vi "Page_Source_Settings_Update_Display.vi"(6 "AB_Build in":refnum<class "AB_Build.lvclass">, 8 "error in (no error)":errorcluster, 9 "ctlReferences":T3, 10 "supportedFunctions":T2, 11 "AB_Source_Container in":refnum<class "AB_Source_Container.lvclass">) -> (0 "error out":errorcluster, 2 "parentApplies":T1, 3 "AB_Source_Container out":refnum<class "AB_Source_Container.lvclass">)   [LabVIEW 2020, in "AB_Source_Container.lvclass"]
uses:
  <vilib>/AppBuilder/AB_Classes/Source/Container/AB_Source_Container.lvclass
  e:/builds/penguin/labview/branches/2020/dev/dist/vi.lib/AppBuilder/AB_Classes/Source/AB_Source.lvclass
  <resource>/Framework/Providers/Builds/AppBuilder/AB_UI_Page_Source_Settings_References.ctl
  <resource>/Framework/Providers/Builds/AppBuilder/AB_UI_Page_Source_Settings_supportedFunctions.ctl
  <vilib>/AppBuilder/AB_Parent_Applies.ctl
  <vilib>/AppBuilder/AB_Classes/Build/AB_Build.lvclass
  <vilib>/AppBuilder/AB_Source_Inclusion.ctl
  <resource>/Framework/Providers/Common/provcom_StringGlobals.vi
  <vilib>/AppBuilder/AB_Classes/Source/AB_Source.lvclass
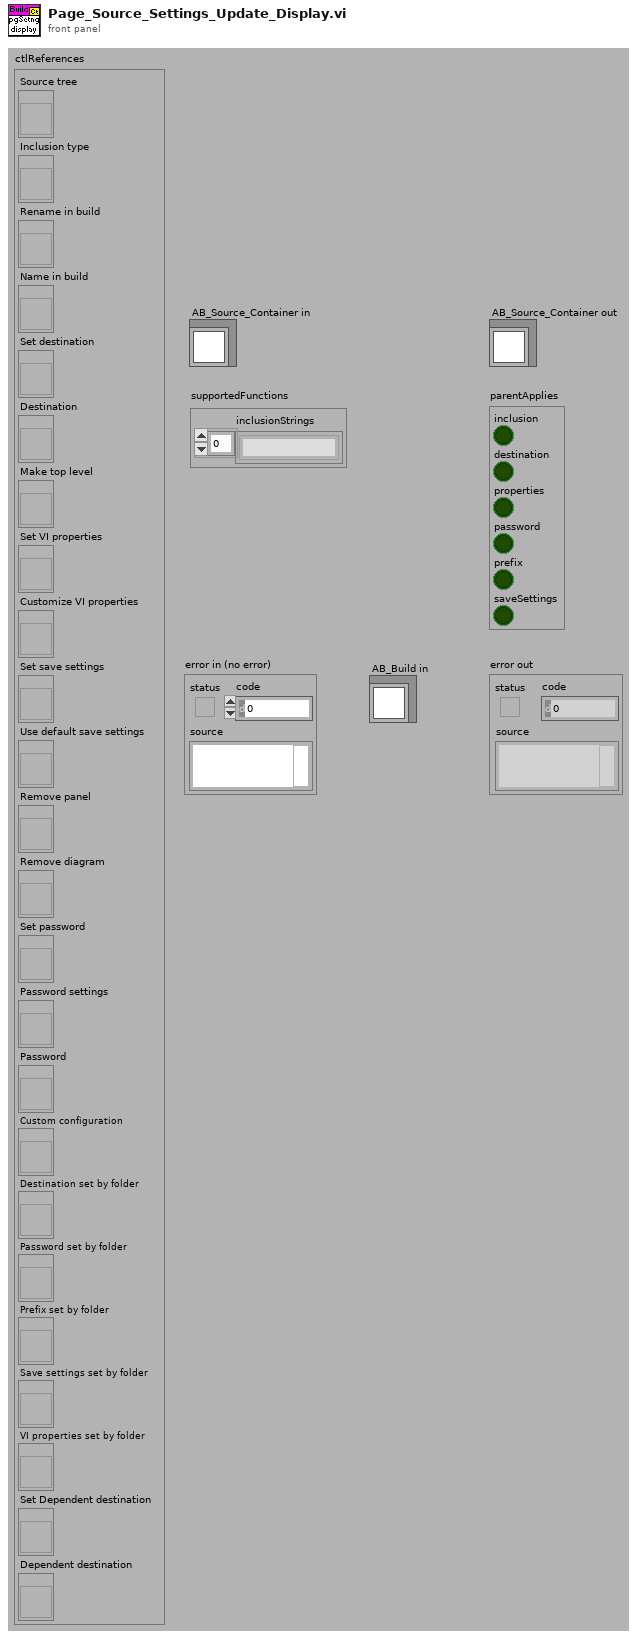
[diagram p1: front panel]
types:
  T1 = typedef "AB_Parent_Applies.ctl" = cluster{"inclusion":bool, "destination":bool, "properties":bool, "password":bool, "prefix":bool, "saveSettings":bool}
  T2 = typedef "AB_UI_Page_Source_Settings_supportedFunctions.ctl" = cluster{"inclusionStrings":string[]}
  T3 = typedef "AB_UI_Page_Source_Settings_References.ctl" = cluster{"Source tree":refnum<vi>, "Inclusion type":refnum<vi>, "Rename in build":refnum<vi>, "Name in build":refnum<vi>, "Set destination":refnum<vi>, "Destination":refnum<vi>, "Make top level":refnum<vi>, "Set VI properties":refnum<vi>, "Customize VI properties":refnum<vi>, "Set save settings":refnum<vi>, "Use default save settings":refnum<vi>, "Remove panel":refnum<vi>, "Remove diagram":refnum<vi>, "Set password":refnum<vi>, "Password settings":refnum<vi>, "Password":refnum<vi>, "Custom configuration":refnum<vi>, "Destination set by folder":refnum<vi>, "Password set by folder":refnum<vi>, "Prefix set by folder":refnum<vi>, "Save settings set by folder":refnum<vi>, "VI properties set by folder":refnum<vi>, "Set Dependent destination":refnum<vi>, "Dependent destination":refnum<vi>}
  T4 = typedef "AB_Build.ctl" = cluster{"buildSpecName":string, "buildSpecDescription":string, "destinations":refnum<class "AB_Destination.lvclass">[], "exclusionOption":T5, "defaultLanguage":string, "supportedLanguages":string[], "excludedDirectories":path[], "buildContext":refnum<vi>, "buildObject":T6, "preview":bool, "programatic":bool, "progressBarEvents":T7, "userLog_Path":path, "preActionID":string, "preAction_Path":path, "postActionID":string, "postAction_Path":path, "eng_checkForBrokenVIs?":bool, "eng_verboseLinkerErrors?":bool, "localDest_Path":path, "targetDest_Path":path, "removeVIObject":u16, "cache":refnum<class "PreviewCache.lvclass">, "use cache":bool, "previewCache_ID":string, "buildCache_ID":string, "eng_TempLocalDest_Path":path, "eng_collectDependencies?":bool, "versionInfo":cluster{"buildVersion":cluster{"major":u16, "minor":u16, "patch":u16, "build":u16}, "autoIncrement":bool}, "eng_enableVIChecksums":bool}
  T5 = typedef "AB_Exclusion_Option.ctl" = cluster{"typedefs":bool, "polymorphicVIs":bool, "unusedLibraryItems":bool, "modifyLibraryFile":bool, "edit-timeDependencies":bool, "inlineVIs":bool, "dependent PPLs":bool, "dependent DLLs":bool}
  T6 = typedef "ItemRef.ctl" = u64
  T7 = typedef "provcom_ProgressBar_Events.ctl" = cluster{"newJob":refnum<user-event>, "newItem":refnum<user-event>, "errorMsg":T8, "cancel":refnum<user-event>}
  T8 = typedef "mxLvBuildError.ctl" = refnum<user-event>
  T9 = typedef "AB_Source.ctl" = cluster{"path":path, "itemID":string, "parentIndex":i32, "sourceInclusion":T10, "destinationIndex":i32, "properties":T11[], "newName":string, "lvfile":bool, "valid":bool, "eng_inBuild":bool, "eng_isNonVILink":bool, "Amalgamation":bool, "Amalgamation Piece":bool, "eng_delimitedName":string, "preventRename":bool}
  T10 = typedef "AB_Source_Inclusion.ctl" = enum16{"IncludeIfReferenced", "Include", "Exclude", "TopLevel"}
  T11 = typedef "AB_Source_Properties.ctl" = cluster{"sourcePropertyType":T12, "value":variant}
  T12 = typedef "AB_Source_Property_Type.ctl" = enum16{"Remove block diagram", "Remove front panel", "Password", "Window has title bar", "Show menu bar", "Show vertical scroll bar", "Show horizontal scroll bar", "Show toolbar", "Show Abort button", "Show fp when called", "Window behavior", "Allow user to close window", "Window run-time position", "Run when opened", "Allow debugging", "Auto error handling", "Generate guard code", "Use stack variables", "Expression folding", "Integer only", "Inline subVI"}
  T13 = typedef "AB_Source_Container.ctl" = cluster{"applyInclusion":bool, "applyDestination":bool, "applyProperties":bool, "applyPassword":bool, "applyPrefix":bool, "applySaveSetttings":bool, "dependentDestinationIndex":i32}
  T14 = enum32{"No password change", "Remove password", "Apply new password"}
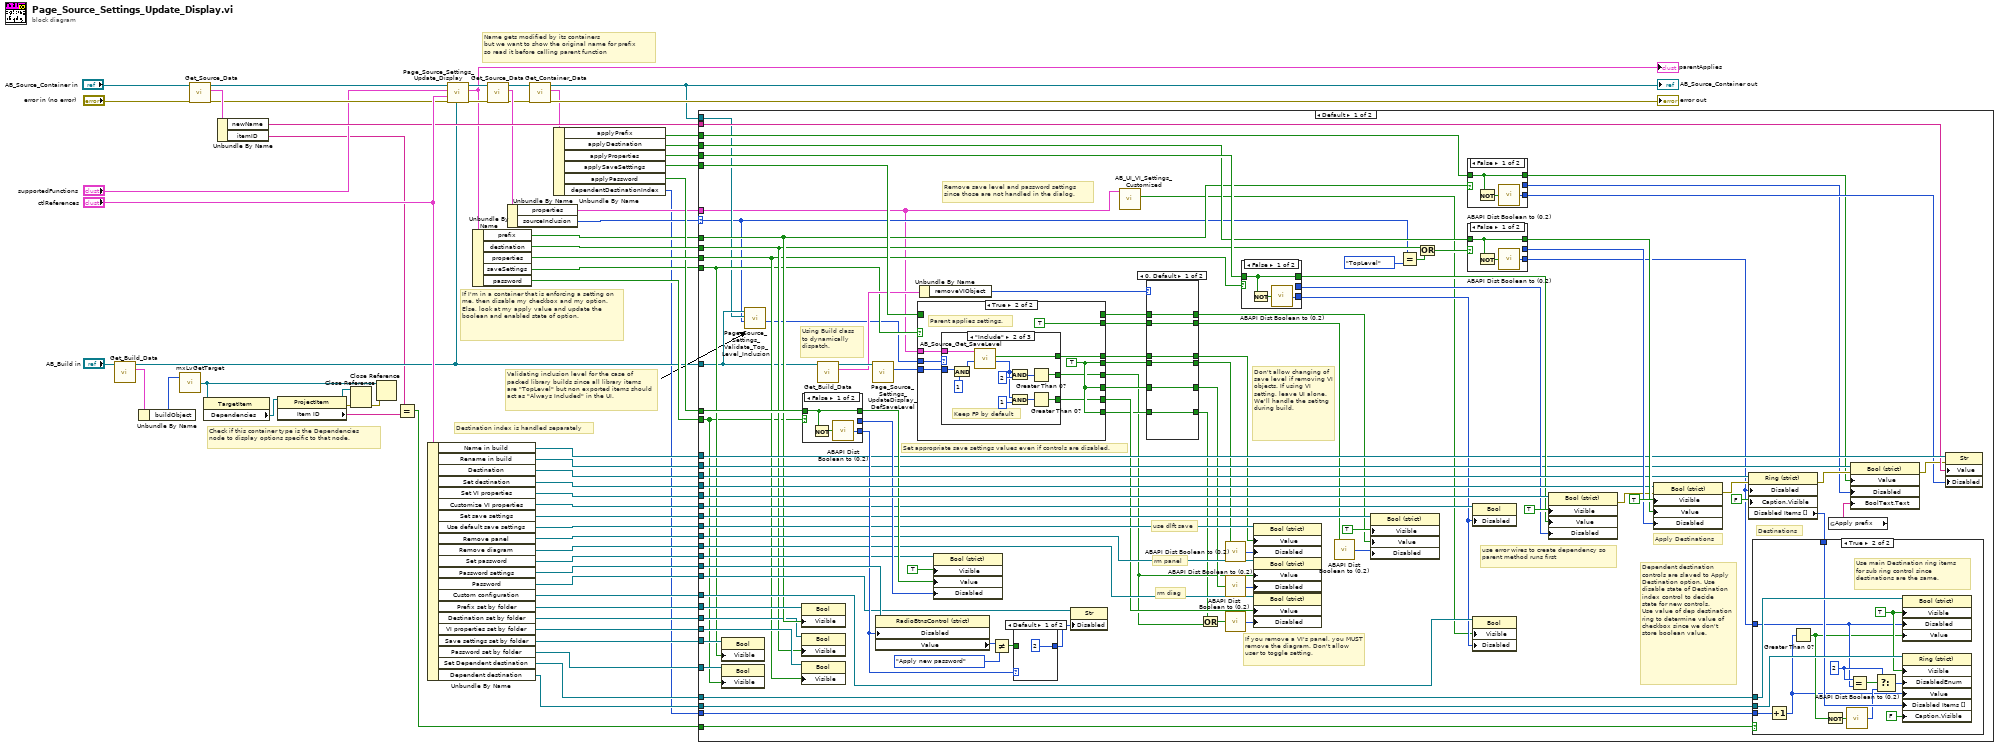
[diagram p0: block diagram]
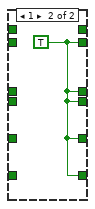
[diagram p3: hidden frame]
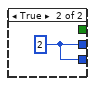
[diagram p4: hidden frame]
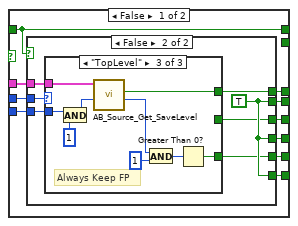
[diagram p5: hidden frame]
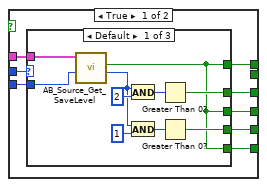
[diagram p6: hidden frame]
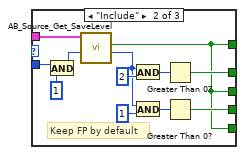
[diagram p7: hidden frame]
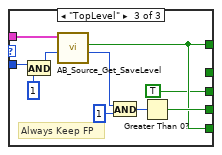
[diagram p8: hidden frame]
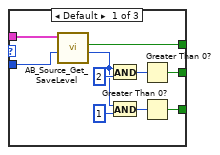
[diagram p9: hidden frame]
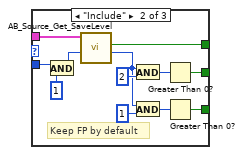
[diagram p10: hidden frame]
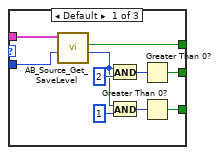
[diagram p11: hidden frame]
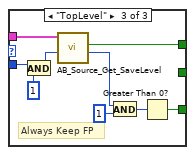
[diagram p12: hidden frame]
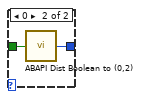
[diagram p13: hidden frame]
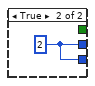
[diagram p14: hidden frame]
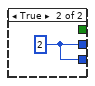
[diagram p15: hidden frame]
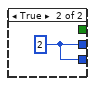
[diagram p16: hidden frame]
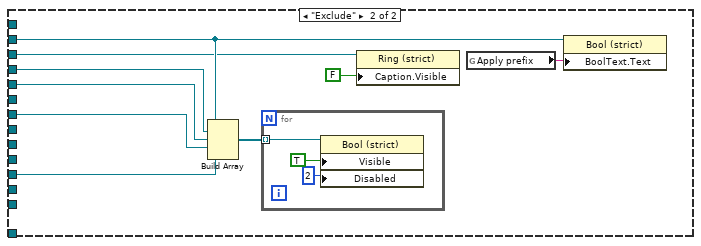
[diagram p17: hidden frame]
diagram:
  # "Check if this container type is the Dependencies node to display options specific to that node."
  # "Validating inclusion level for the case of packed library builds since all library items are \"TopLevel\" but non exported items should act as \"Always Included\" in the UI."
  # "If I'm in a container that is enforcing a setting on me, then disable my checkbox and my option.\nElse, look at my apply value and update the boolean and enabled state of option."
  # "Name gets modified by its containers\nbut we want to show the original name for prefix\nso read it before calling parent function"
  # "Destination index is handled separately"
  n1 = call <vilib>:"Get_Build_Data.vi"("Class in"="AB_Build in") -> ("data"=w12:T4, "Class out"=w13:refnum<class "AB_Build.lvclass">)  [unwired: 8 in, 1 out]
  n2 = Unbundle By Name(w12) -> ("buildObject"=w6:T6)
  n3 = call <resource>:"mxLvGetTarget.vi"("Item"=w6) -> ("Target"=w7:refnum<vi>)  [unwired: 1 in, 2 out]
  n4 = call <vilib>:"Get_Source_Data.vi"("error in (no error)"="error in (no error)", "Class in"="AB_Source_Container in") -> ("error out"=w47:errorcluster, "data"=w51:T9, "Class out"=w49:refnum<class "AB_Source_Container.lvclass">)  [unwired: 7 in]
  n5 = property class="TargetItem"(reference=w7) -> ("Dependencies"=w11:refnum<vi>)  [unwired: 1 in, 2 out]
  n6 = Unbundle By Name(w51) -> ("newName"=w50:string, "itemID"=w4:string)
  n7 = property class="ProjectItem"(reference=w11) -> (reference out=w9:refnum<vi>, error out=w10:errorcluster, "Item ID"=w5:string)  [unwired: 1 in]
  n8 = Close Reference(reference=w9, error in (no error)=w10) -> (error out=w8:errorcluster)
  n9 = Close Reference(reference=w7, error in (no error)=w8) -> ()  [unwired: 1 out]
  n10 = Equal?(x=w4, y=w5) -> (x = y?=w3:bool)
  n11 = Unbundle By Name("ctlReferences") -> ("Name in build"=w53:refnum<vi>, "Rename in build"=w54:refnum<vi>, "Destination"=w59:refnum<vi>, "Set destination"=w61:refnum<vi>, "Set VI properties"=w60:refnum<vi>, "Customize VI properties"=w34:refnum<vi>, "Set save settings"=w33:refnum<vi>, "Use default save settings"=w32:refnum<vi>, "Remove panel"=w28:refnum<vi>, "Remove diagram"=w27:refnum<vi>, "Set password"=w35:refnum<vi>, "Password settings"=w62:refnum<vi>, "Password"=w58:refnum<vi>, "Custom configuration"=w23:refnum<vi>, "Prefix set by folder"=w22:refnum<vi>, "Destination set by folder"=w21:refnum<vi>, "VI properties set by folder"=w20:refnum<vi>, "Save settings set by folder"=w19:refnum<vi>, "Password set by folder"=w18:refnum<vi>, "Set Dependent destination"=w16:refnum<vi>, "Dependent destination"=w15:refnum<vi>)
  n12 = call-parent "Page_Source_Settings_Update_Display.vi"("AB_Build in"=w13, "error in (no error)"=w47, "ctlReferences"="ctlReferences", "supportedFunctions"="supportedFunctions", "AB_Source in"=w49) -> ("error out"=w43:errorcluster, "parentApplies"=w1:T1, "AB_Source out"=w45:refnum<class "AB_Source_Container.lvclass">)  [unwired: 4 in]
  "parentApplies" <- w1
  n13 = Unbundle By Name(w1) -> ("prefix"=w24:bool, "destination"=w57:bool, "properties"=w56:bool, "saveSettings"=w30:bool, "password"=w55:bool)
  n14 = call <vilib>:"Get_Source_Data.vi"("error in (no error)"=w43, "Class in"=w45) -> ("error out"=w42:errorcluster, "data"=w46:T9, "Class out"=w44:refnum<class "AB_Source_Container.lvclass">)  [unwired: 7 in]
  n15 = Unbundle By Name(w46) -> ("properties"=w29:T11[], "sourceInclusion"=w25:T10)
  n16 = call <vilib>:"Get_Container_Data.vi"("error in (no error)"=w42, "Class in"=w44) -> ("error out"=→"error out":errorcluster, "data"=w40:T13, "Class out"=w17:refnum<class "AB_Source_Container.lvclass">)  [unwired: 7 in]
  "AB_Source_Container out" <- w17
  n17 = Unbundle By Name(w40) -> ("applyPrefix"=w36:bool, "applyDestination"=w37:bool, "applyProperties"=w38:bool, "applySaveSetttings"=w26:bool, "applyPassword"=w39:bool, "dependentDestinationIndex"=w2:i32)
  n18 = case shown="Default" w25 {
    selector: w25 -> [w73 _]
    tunnel: w62 -> [w156 _]
    tunnel: w61 -> [w152 w329]
    tunnel: w60 -> [w149 w330]
    tunnel: w59 -> [w148 w324]
    tunnel: w58 -> [w141 _]
    tunnel: w57 -> [w85 _]
    tunnel: w56 -> [w84 _]
    tunnel: w55 -> [w80 _]
    tunnel: w54 -> [w133 w328]
    tunnel: w53 -> [w132 _]
    tunnel: w50 -> [w131 _]
    tunnel: w39 -> [w130 _]
    tunnel: w38 -> [w129 _]
    tunnel: w37 -> [w128 _]
    tunnel: w36 -> [w108 _]
    tunnel: w35 -> [w123 w327]
    tunnel: w34 -> [w122 _]
    tunnel: w33 -> [w120 w331]
    tunnel: w32 -> [w119 _]
    tunnel: w30 -> [w81 _]
    tunnel: w29 -> [w71 _]
    tunnel: w28 -> [w118 _]
    tunnel: w27 -> [w117 _]
    tunnel: w26 -> [w113 _]
    tunnel: w24 -> [w88 _]
    tunnel: w13 -> [w75 _]
    tunnel: w23 -> [w91 _]
    tunnel: w22 -> [w89 _]
    tunnel: w21 -> [w87 _]
    tunnel: w20 -> [w86 _]
    tunnel: w19 -> [w83 _]
    tunnel: w18 -> [w82 _]
    tunnel: w17 -> [w74 _]
    tunnel: w16 -> [w68 _]
    tunnel: w15 -> [w67 _]
    tunnel: w3 -> [w69 _]
    tunnel: w2 -> [w65 _]
    frame Default {
      # "Dependent destination controls are slaved to Apply Destination option. Use disable state of Destination index control to decide state for new controls. \nUse value of dep destination ring to determine value of checkbox since we don't store boolean value."
      # "Apply Destinations"
      # "Destinations"
      # "Remove save level and password settings since those are not handled in the dialog."
      # "Set appropriate save settings values even if controls are disabled."
      # "use dlft save"
      # "rm diag"
      # "rm panel"
      # "If you remove a VI's panel, you MUST remove the diagram. Don't allow user to toggle setting."
      # "Don't allow changing of save level if removing VI objects. If using VI setting, leave UI alone. We'll handle the setitng during build."
      # "Using Build class to dynamically dispatch."
      # "use error wires to create dependency so parent method runs first"
      n19 = property class="Bool"(reference=w83, "Visible"=w81) -> ()  [unwired: 1 in, 2 out]
      n20 = property class="Bool"(reference=w82, "Visible"=w80) -> ()  [unwired: 1 in, 2 out]
      n21 = call-dynamic "Page_Source_Settings_Validate_Top_Level_Inclusion.vi"("sourceInclusion in"=w73, "AB_Source in"=w74, "AB_Build in"=w75) -> ("sourceInclusion out"=w72:T10)  [unwired: 6 in, 2 out]
      n22 = property class="Bool"(reference=w89, "Visible"=w88) -> ()  [unwired: 1 in, 2 out]
      n23 = property class="Bool"(reference=w87, "Visible"=w85) -> ()  [unwired: 1 in, 2 out]
      n24 = property class="Bool"(reference=w86, "Visible"=w84) -> ()  [unwired: 1 in, 2 out]
      n25 = case shown="False" w80 {
        tunnel: [_ w315] -> w144
        tunnel: [w314 _] -> w145
        tunnel: w130 -> [w314 _]
        tunnel: [w312 w315] -> w142
        frame False {
          n26 = Not(x=w314) -> (.not. x?=w313:bool)
          n27 = call <vilib>:"ABAPI Dist Boolean to (0,2).vi"("Boolean"=w313) -> ("0, 2"=w312:u8)  [unwired: 4 in]
        }
        frame True {
          w315 = u8 2 ("Disabled")
        }
      }
      n28 = call <vilib>:"Get_Build_Data.vi"("Class in"=w75) -> ("data"=w104:T4, "Class out"=w105:refnum<class "AB_Build.lvclass">)  [unwired: 8 in, 1 out]
      n29 = call-dynamic "Page_Source_Settings_UpdateDisplay_DefSaveLevel.vi"("AB_Build in"=w105) -> ("defaultSaveLevel"=w106:u32)  [unwired: 8 in, 2 out]
      n30 = property class="RadioBtnsControl (strict)"(reference=w156, "Disabled"=w142) -> ("Value"=w140:T14)  [unwired: 1 in, 2 out]
      n31 = case shown="True" w81 {
        tunnel: w106 -> [w191 w271]
        tunnel: w71 -> [w190 w270]
        tunnel: [w188 w273] -> w102
        tunnel: [w187 w277] -> w101
        tunnel: [w186 w275] -> w79
        tunnel: [w185 w277] -> w100
        tunnel: [w184 w274] -> w114
        tunnel: [w183 w277] -> w99
        tunnel: w113 -> [w182 _]
        tunnel: w72 -> [w189 w272]
        tunnel: [w182 _] -> w95
        tunnel: [_ TRUE] -> w94
        frame False {
          n32 = case shown="False" w182 {
            tunnel: w189 -> [w192 w234]
            tunnel: w190 -> [w199 w233]
            tunnel: [w198 w235] -> w188
            tunnel: [_ w238] -> w187
            tunnel: [w197 w238] -> w185
            tunnel: [w196 w238] -> w183
            tunnel: w191 -> [w195 w232]
            tunnel: [w194 w237] -> w186
            tunnel: [w193 w236] -> w184
            frame True {
              n33 = case shown="Default" w192 {
                tunnel: w199 -> [w209 w221 w231]
                tunnel: [w200 w210 w227] -> w198
                tunnel: [w200 w210 TRUE] -> w197
                tunnel: [w200 w210 w227] -> w196
                tunnel: w195 -> [w208 w216 w225]
                tunnel: [w205 w212 _] -> w194
                tunnel: [w201 w218 w228] -> w193
                frame Default {
                  n34 = call <vilib>:"AB_Source_Get_SaveLevel.vi"("defaultSaveLevel"=w208, "sourceProperties in"=w209) -> ("saveLevel out"=w202:u32, "useDefault"=w200:bool)  [unwired: 6 in, 2 out]
                  n35 = And(x=w202, y=u32 2) -> (x .and. y?=w206:u32)
                  n36 = And(x=w202, y=u32 1) -> (x .and. y?=w204:u32)
                  n37 = Greater Than 0?(x=w206) -> (x > 0?=w205:bool)
                  n38 = Greater Than 0?(x=w204) -> (x > 0?=w201:bool)
                }
                frame "Include" {
                  # "Keep FP by default"
                  n39 = And(x=w216, y=u32 1 ("defaultSaveLevel")) -> (x .and. y?=w215:u32)
                  n40 = call <vilib>:"AB_Source_Get_SaveLevel.vi"("defaultSaveLevel"=w215, "sourceProperties in"=w221) -> ("saveLevel out"=w211:u32, "useDefault"=w210:bool)  [unwired: 6 in, 2 out]
                  n41 = And(x=w211, y=u32 2) -> (x .and. y?=w213:u32)
                  n42 = And(x=w211, y=u32 1) -> (x .and. y?=w220:u32)
                  n43 = Greater Than 0?(x=w213) -> (x > 0?=w212:bool)
                  n44 = Greater Than 0?(x=w220) -> (x > 0?=w218:bool)
                }
                frame "TopLevel" {
                  # "Always Keep FP"
                  n45 = And(x=w225, y=u32 1 ("defaultSaveLevel")) -> (x .and. y?=w224:u32)
                  n46 = call <vilib>:"AB_Source_Get_SaveLevel.vi"("defaultSaveLevel"=w224, "sourceProperties in"=w231) -> ("saveLevel out"=w223:u32, "useDefault"=w227:bool)  [unwired: 6 in, 2 out]
                  n47 = And(x=w223, y=u32 1) -> (x .and. y?=w230:u32)
                  n48 = Greater Than 0?(x=w230) -> (x > 0?=w228:bool)
                }
              }
            }
            frame False {
              w238 = TRUE
              n49 = case shown="\"TopLevel\"" w234 {
                tunnel: w233 -> [w248 w260 w269]
                tunnel: [w239 w249 w261] -> w235
                tunnel: w232 -> [w247 w255 w264]
                tunnel: [w244 w251 _] -> w237
                tunnel: [w240 w257 w266] -> w236
                frame Default {
                  n50 = call <vilib>:"AB_Source_Get_SaveLevel.vi"("defaultSaveLevel"=w247, "sourceProperties in"=w248) -> ("saveLevel out"=w241:u32, "useDefault"=w239:bool)  [unwired: 6 in, 2 out]
                  n51 = And(x=w241, y=u32 2) -> (x .and. y?=w245:u32)
                  n52 = And(x=w241, y=u32 1) -> (x .and. y?=w243:u32)
                  n53 = Greater Than 0?(x=w245) -> (x > 0?=w244:bool)
                  n54 = Greater Than 0?(x=w243) -> (x > 0?=w240:bool)
                }
                frame "Include" {
                  # "Keep FP by default"
                  n55 = And(x=w255, y=u32 1 ("defaultSaveLevel")) -> (x .and. y?=w254:u32)
                  n56 = call <vilib>:"AB_Source_Get_SaveLevel.vi"("defaultSaveLevel"=w254, "sourceProperties in"=w260) -> ("saveLevel out"=w250:u32, "useDefault"=w249:bool)  [unwired: 6 in, 2 out]
                  n57 = And(x=w250, y=u32 2) -> (x .and. y?=w252:u32)
                  n58 = And(x=w250, y=u32 1) -> (x .and. y?=w259:u32)
                  n59 = Greater Than 0?(x=w252) -> (x > 0?=w251:bool)
                  n60 = Greater Than 0?(x=w259) -> (x > 0?=w257:bool)
                }
                frame "TopLevel" {
                  # "Always Keep FP"
                  n61 = And(x=w264, y=u32 1 ("defaultSaveLevel")) -> (x .and. y?=w263:u32)
                  n62 = call <vilib>:"AB_Source_Get_SaveLevel.vi"("defaultSaveLevel"=w263, "sourceProperties in"=w269) -> ("saveLevel out"=w262:u32, "useDefault"=w261:bool)  [unwired: 6 in, 2 out]
                  n63 = And(x=w262, y=u32 1) -> (x .and. y?=w268:u32)
                  n64 = Greater Than 0?(x=w268) -> (x > 0?=w266:bool)
                }
              }
            }
          }
        }
        frame True {
          w277 = TRUE
          # "Parent applies settings."
          n65 = case shown="\"Include\"" w272 {
            tunnel: w270 -> [w287 w299 w308]
            tunnel: [w278 w288 w300] -> w273
            tunnel: w271 -> [w286 w294 w303]
            tunnel: [w283 w290 _] -> w275
            tunnel: [w279 w296 w305] -> w274
            frame Default {
              n66 = call <vilib>:"AB_Source_Get_SaveLevel.vi"("defaultSaveLevel"=w286, "sourceProperties in"=w287) -> ("saveLevel out"=w280:u32, "useDefault"=w278:bool)  [unwired: 6 in, 2 out]
              n67 = And(x=w280, y=u32 2) -> (x .and. y?=w284:u32)
              n68 = And(x=w280, y=u32 1) -> (x .and. y?=w282:u32)
              n69 = Greater Than 0?(x=w284) -> (x > 0?=w283:bool)
              n70 = Greater Than 0?(x=w282) -> (x > 0?=w279:bool)
            }
            frame "Include" {
              # "Keep FP by default"
              n71 = And(x=w294, y=u32 1 ("defaultSaveLevel")) -> (x .and. y?=w293:u32)
              n72 = call <vilib>:"AB_Source_Get_SaveLevel.vi"("defaultSaveLevel"=w293, "sourceProperties in"=w299) -> ("saveLevel out"=w289:u32, "useDefault"=w288:bool)  [unwired: 6 in, 2 out]
              n73 = And(x=w289, y=u32 2) -> (x .and. y?=w291:u32)
              n74 = And(x=w289, y=u32 1) -> (x .and. y?=w298:u32)
              n75 = Greater Than 0?(x=w291) -> (x > 0?=w290:bool)
              n76 = Greater Than 0?(x=w298) -> (x > 0?=w296:bool)
            }
            frame "TopLevel" {
              # "Always Keep FP"
              n77 = And(x=w303, y=u32 1 ("defaultSaveLevel")) -> (x .and. y?=w302:u32)
              n78 = call <vilib>:"AB_Source_Get_SaveLevel.vi"("defaultSaveLevel"=w302, "sourceProperties in"=w308) -> ("saveLevel out"=w301:u32, "useDefault"=w300:bool)  [unwired: 6 in, 2 out]
              n79 = And(x=w301, y=u32 1) -> (x .and. y?=w307:u32)
              n80 = Greater Than 0?(x=w307) -> (x > 0?=w305:bool)
            }
          }
        }
      }
      n81 = Unbundle By Name(w104) -> ("removeVIObject"=w103:u16)
      n82 = property class="Bool (strict)"(reference=w123, "Visible"=TRUE, "Value"=w145, "Disabled"=w144) -> ()  [unwired: 1 in, 2 out]
      n83 = Not Equal?(x=w140, y=T14."Apply new password") -> (x != y?=w138:bool)
      n84 = case shown="Default" w142 {
        tunnel: w138 -> [_ w311]
        tunnel: [u8 2 ("0, 2") w310] -> w137
        frame Default {
        }
        frame 0 {
          n85 = call <vilib>:"ABAPI Dist Boolean to (0,2).vi"("Boolean"=w311) -> ("0, 2"=w310:u8)  [unwired: 4 in]
        }
      }
      n86 = property class="Str"(reference=w141, "Disabled"=w137) -> ()  [unwired: 1 in, 2 out]
      n87 = call <resource>:"AB_UI_VI_Settings_Customized.vi"("sourceProperties in"=w71) -> ("customized"=w70:bool)  [unwired: 9 in, 1 out]
      n88 = case shown="0, Default" w103 {
        tunnel: w102 -> [w176 _]
        tunnel: w101 -> [w175 _]
        tunnel: w100 -> [w174 _]
        tunnel: w99 -> [w173 _]
        tunnel: [w176 w177] -> w98
        tunnel: [w175 w177] -> w97
        tunnel: [w174 w177] -> w96
        tunnel: [w173 w177] -> w78
        tunnel: w95 -> [w172 _]
        tunnel: w94 -> [w171 _]
        tunnel: [w172 _] -> w93
        tunnel: [w171 w177] -> w92
        frame 0, Default {
        }
        frame 1 {
          w177 = TRUE ("useDefault")
        }
      }
      n89 = Or(x=w78, y=w79) -> (x .or. y?=w77:bool)
      n90 = call <vilib>:"ABAPI Dist Boolean to (0,2).vi"("Boolean"=w97) -> ("0, 2"=w116:u8)  [unwired: 4 in]
      n91 = call <vilib>:"ABAPI Dist Boolean to (0,2).vi"("Boolean"=w96) -> ("0, 2"=w115:u8)  [unwired: 4 in]
      n92 = call <vilib>:"ABAPI Dist Boolean to (0,2).vi"("Boolean"=w77) -> ("0, 2"=w76:u8)  [unwired: 4 in]
      n93 = case shown="False" w84 {
        tunnel: [_ w319] -> w146
        tunnel: [w318 _] -> w147
        tunnel: w129 -> [w318 _]
        tunnel: [w316 w319] -> w90
        frame False {
          n94 = Not(x=w318) -> (.not. x?=w317:bool)
          n95 = call <vilib>:"ABAPI Dist Boolean to (0,2).vi"("Boolean"=w317) -> ("0, 2"=w316:u8)  [unwired: 4 in]
        }
        frame True {
          w319 = u8 2 ("Disabled")
        }
      }
      n96 = property class="Bool (strict)"(reference=w119, "Value"=w98, "Disabled"=w116) -> ()  [unwired: 1 in, 2 out]
      n97 = property class="Bool (strict)"(reference=w118, "Value"=w79, "Disabled"=w115) -> ()  [unwired: 1 in, 2 out]
      n98 = property class="Bool (strict)"(reference=w117, "Value"=w114, "Disabled"=w76) -> ()  [unwired: 1 in, 2 out]
      n99 = call <vilib>:"ABAPI Dist Boolean to (0,2).vi"("Boolean"=w92) -> ("0, 2"=w112:u8)  [unwired: 4 in]
      n100 = property class="Bool (strict)"(reference=w120, "Visible"=TRUE, "Value"=w93, "Disabled"=w112) -> ()  [unwired: 1 in, 2 out]
      n101 = Equal?(x=w73, y=AB_Source_Inclusion."TopLevel" ("x")) -> (x = y?=w135:bool)
      n102 = Or(x=w85, y=w135) -> (x .or. y?=w134:bool)
      n103 = case shown="False" w88 {
        tunnel: [_ w181] -> w109
        tunnel: [w180 _] -> w107
        tunnel: w108 -> [w180 _]
        tunnel: [w178 w181] -> w110
        frame False {
          n104 = Not(x=w180) -> (.not. x?=w179:bool)
          n105 = call <vilib>:"ABAPI Dist Boolean to (0,2).vi"("Boolean"=w179) -> ("0, 2"=w178:u8)  [unwired: 4 in]
        }
        frame True {
          w181 = u8 2 ("Disabled")
        }
      }
      n106 = case shown="False" w134 {
        tunnel: [_ w323] -> w154
        tunnel: [w322 _] -> w153
        tunnel: w128 -> [w322 _]
        tunnel: [w320 w323] -> w64
        frame False {
          n107 = Not(x=w322) -> (.not. x?=w321:bool)
          n108 = call <vilib>:"ABAPI Dist Boolean to (0,2).vi"("Boolean"=w321) -> ("0, 2"=w320:u8)  [unwired: 4 in]
        }
        frame True {
          w323 = u8 2 ("Disabled")
        }
      }
      n109 = property class="Bool"(reference=w122, "Disabled"=w90) -> ()  [unwired: 1 in, 2 out]
      n110 = property class="Bool"(reference=w91, "Visible"=w70, "Disabled"=w90) -> ()  [unwired: 1 in, 2 out]
      n111 = property class="Bool (strict)"(reference=w149, "Visible"=TRUE, "Value"=w147, "Disabled"=w146) -> (error out=w127:errorcluster)  [unwired: 1 in, 1 out]
      n112 = property class="Bool (strict)"(reference=w152, error in=w127, "Visible"=TRUE, "Value"=w153, "Disabled"=w154) -> (error out=w126:errorcluster)  [unwired: 1 out]
      n113 = property class="Ring (strict)"(reference=w148, error in=w126, "Disabled"=w64, "Caption.Visible"=FALSE) -> (error out=w125:errorcluster, "Disabled Items []"=w66:i32[])  [unwired: 1 out]
      n114 = case shown="True" w69 {
        tunnel: w68 -> [_ w170]
        tunnel: w67 -> [_ w169]
        tunnel: w64 -> [_ w161]
        tunnel: w66 -> [_ w167]
        tunnel: w65 -> [_ w158]
        frame False {
        }
        frame True {
          w162 = u8 2 ("y")
          w166 = TRUE ("Visible")
          # "Use main Destination ring items for sub ring control since destinations are the same."
          n115 = Increment(x=w158) -> (x+1=w157:i32)
          n116 = Greater Than 0?(x=w157) -> (x > 0?=w159:bool)
          n117 = Not(x=w159) -> (.not. x?=w163:bool)
          n118 = call <vilib>:"ABAPI Dist Boolean to (0,2).vi"("Boolean"=w163) -> ("0, 2"=w160:u8)  [unwired: 4 in]
          n119 = Equal?(x=w162, y=w161) -> (x = y?=w165:bool)
          n120 = Select(t=w162, s=w165, f=w160) -> (s? t:f=w164:u8)
          n121 = property class="Bool (strict)"(reference=w170, "Visible"=w166, "Disabled"=w161, "Value"=w159) -> ()  [unwired: 1 in, 2 out]
          n122 = property class="Ring (strict)"(reference=w169, "Visible"=w166, "DisabledEnum"=w164, "Value"=w157, "Disabled Items []"=w167, "Caption.Visible"=FALSE) -> ()  [unwired: 1 in, 2 out]
        }
      }
      n123 = global read "provcom_StringGlobals.vi" "Apply prefix"() -> (w111:string)
      n124 = property class="Bool (strict)"(reference=w133, error in=w125, "Value"=w107, "Disabled"=w109, "BoolText.Text"=w111) -> (error out=w124:errorcluster)  [unwired: 1 out]
      n125 = property class="Str"(reference=w132, error in=w124, "Value"=w131, "Disabled"=w110) -> ()  [unwired: 2 out]
    }
    frame "Exclude" {
      n126 = Build Array(w328, w329, w330, w331, w327) -> (w326:refnum<vi>[])
      n127 = for {
        tunnel: w326 -> [w334] mode=indexing
        n128 = property class="Bool (strict)"(reference=w334, "Visible"=TRUE, "Disabled"=u8 2) -> ()  [unwired: 1 in, 2 out]
      }
      n129 = property class="Ring (strict)"(reference=w324, "Caption.Visible"=FALSE) -> ()  [unwired: 1 in, 2 out]
      n130 = global read "provcom_StringGlobals.vi" "Apply prefix"() -> (w332:string)
      n131 = property class="Bool (strict)"(reference=w328, "BoolText.Text"=w332) -> ()  [unwired: 1 in, 2 out]
    }
  }
